vi "AssertTargetsHaveCorrectVeriStandVersion.vi"(8 "error in (no error)":errorcluster, 11 "targets":string[](array[string])=["localhost"]) -> (0 "error out":errorcluster)   [LabVIEW 2016, in "VeriStandTestUtilities.lvlib"]
uses:
  VeriStandTestUtilities.lvlib
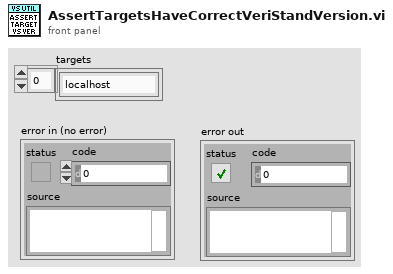
[diagram p1: front panel]
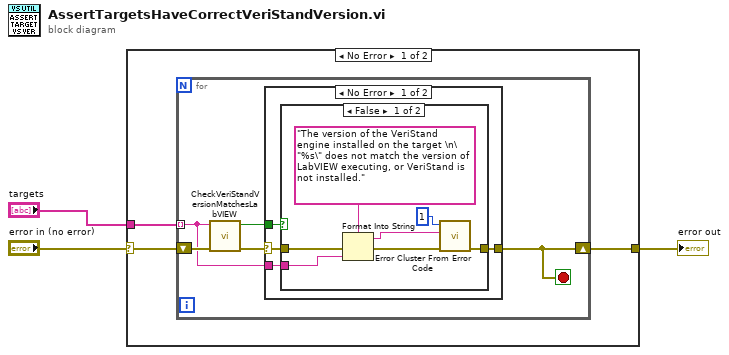
[diagram p0: block diagram]
diagram:
  n1 = case shown="No Error" "error in (no error)" {
    selector: "error in (no error)" -> [w5 w25]
    tunnel: [w6 w25] -> w3
    tunnel: "targets" -> [w4 _]
    frame No Error {
      n2 = for {
        tunnel: w4 -> [w8] mode=indexing
        shift-right: [w7] -> w6
        shift-left: w5 -> [w10]
        stop <- w7 stop-if-true
        n3 = call "CheckVeriStandVersionMatchesLabVIEW.vi"("error in (no error)"=w10, "Target (localhost)"=w8) -> ("error out"=w9:errorcluster, "versions match?"=w11:bool)  [unwired: 8 in]
        n4 = case shown="No Error" w9 {
          selector: w9 -> [w14 w24]
          tunnel: w11 -> [w15 _]
          tunnel: w8 -> [w13 _]
          tunnel: [w12 w24] -> w7
          frame No Error {
            n5 = case shown="False" w15 {
              tunnel: [w21 w23] -> w12
              tunnel: w14 -> [w18 w23]
              tunnel: w13 -> [w20 _]
              frame False {
                n6 = Format Into String(format string="The version of the VeriStand engine installed on the target \n\"%s\" does not match the version of LabVIEW executing, or VeriStand is not installed.", error in=w18, w20) -> (resulting string=w16:string, error out=w17:errorcluster)  [unwired: 1 in]
                n7 = call <vilib>:"Error Cluster From Error Code.vi"("error in (no error)"=w17, "error message (\"\")"=w16, "error code (0)"=1) -> ("error out"=w21:errorcluster)  [unwired: 6 in]
              }
              frame True {
              }
            }
          }
          frame Error {
          }
        }
      }
    }
    frame Error {
    }
  }
  "error out" <- w3
